vi "TTA_MATLAB_Tile_RFPAL_Reset.vi"(0 "Channels":string[](array[combo]), 5 "Mode":enum16{"SoftReset", "HardReset"}(ring), 11 "error in":errorcluster) -> (4 "Success":bool, 6 "TileSuccessComm":bool[](array[boolean]), 8 "TileSuccessOp":bool[](array[boolean]), 15 "error out":errorcluster)   [LabVIEW 2016]
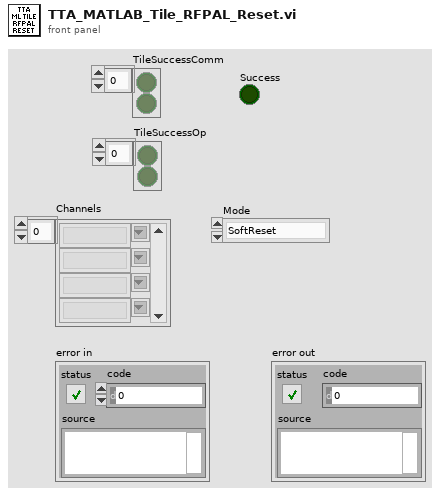
[diagram p1: front panel]
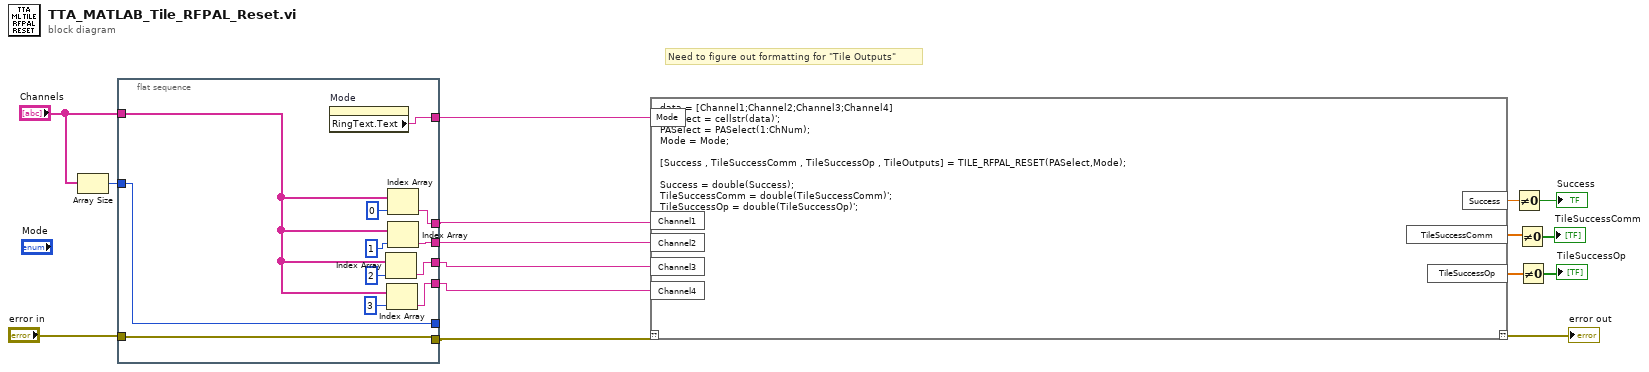
[diagram p0: block diagram]
diagram:
  # "Need to figure out formatting for \"Tile Outputs\""
  n1 = Array Size(array="Channels") -> (size(s)=w8:i32)
  n2 = flat-sequence {
    tunnel: "error in" -> [w28]
    tunnel: [w27] -> w6
    tunnel: w8 -> [w21]
    tunnel: [w28] -> w9
    tunnel: "Channels" -> [w20]
    tunnel: [w24] -> w5
    tunnel: [w22] -> w4
    tunnel: [w21] -> _
    tunnel: [w18] -> w3
    tunnel: [w17] -> w11
    frame #0 {
      n3 = property on="Mode" class="Enum (strict)"() -> ("RingText.Text"=w17:string)  [unwired: 2 in, 2 out]
      n4 = Index Array(array=w20, index=2) -> (element=w22:string)
      n5 = Index Array(array=w20, index=3) -> (element=w18:string)
      n6 = Index Array(array=w20, index=0) -> (element=w27:string)
      n7 = Index Array(array=w20, index=1) -> (element=w24:string)
    }
  }
  n8 = script code="data = [Channel1;Channel2;Channel3;Channel4]\nPASelect = cellstr(data)';\nPASelect = PASelect(1:ChNum);\nMode = Mode;\n\n[Success , TileSuccessComm , TileSuccessOp , TileOutputs] = TILE_RFPAL_RESET(PASelect,Mode);\n\nSuccess = double(Success);\nTileSuccessComm = double(TileSuccessComm)';\nTileSuccessOp = double(TileSuccessOp)';"("??"=w9, "Channel1"=w6, "Mode"=w11, "Channel2"=w5, "Channel3"=w4, "Channel4"=w3) -> ("??"=→"error out":errorcluster, "Success"=w15:dbl, "TileSuccessComm"=w13:dbl[], "TileSuccessOp"=w12:dbl[])
  n9 = Not Equal To 0?(x=w15) -> (x != 0?=→"Success":bool)
  n10 = Not Equal To 0?(x=w13) -> (x != 0?=→"TileSuccessComm":bool[])
  n11 = Not Equal To 0?(x=w12) -> (x != 0?=→"TileSuccessOp":bool[])
